vi "放置控件.vi"(8 "error in (no error)":errorcluster caption="错误输入（无错误）", 11 "程序响应 输入":refnum<class "程序响应.lvclass">) -> (0 "error out":errorcluster caption="错误输出", 3 "程序响应 输出":refnum<class "程序响应.lvclass">)   [LabVIEW 2018, in "程序响应.lvlib" / "程序响应.lvclass"]
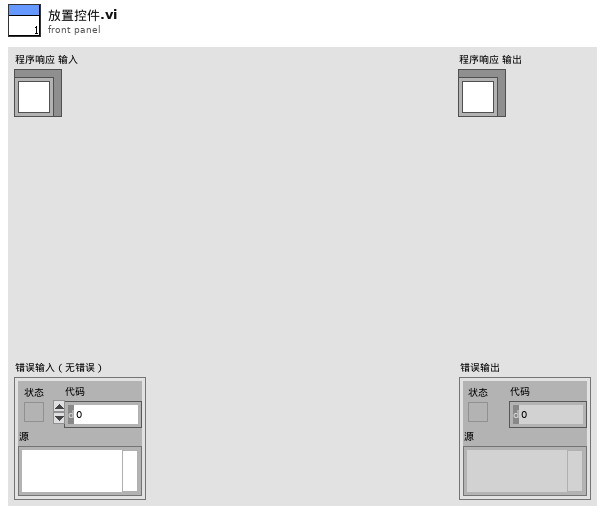
[diagram p1: front panel]
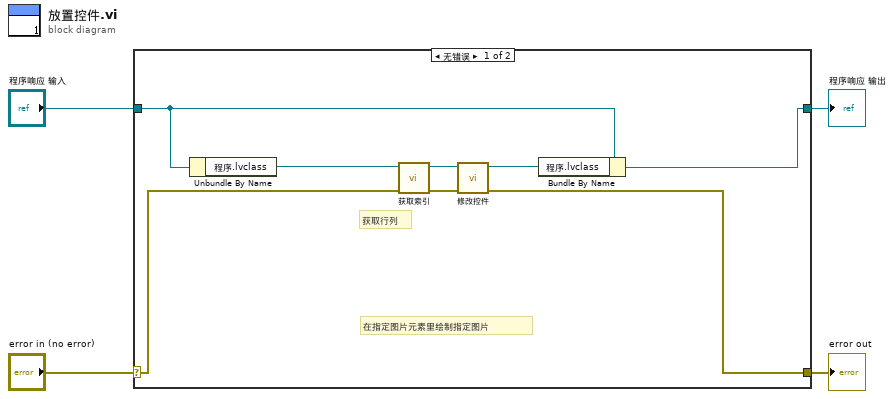
[diagram p0: block diagram]
diagram:
  n1 = case shown="无错误" "error in (no error)" {
    selector: "error in (no error)" -> [w5 w14]
    tunnel: [w9 w14] -> w3
    tunnel: [w11 w13] -> w1
    tunnel: "程序响应 输入" -> [w12 w13]
    frame No Error {
      # "在指定图片元素里绘制指定图片"
      # "获取行列"
      n2 = Unbundle By Name(w12) -> ("程序.lvclass"=w6:refnum<class "程序.lvclass">)
      n3 = call-dynamic "获取索引.vi"("error in (no error)"=w5, "程序 输入"=w6) -> ("error out"=w7:errorcluster, "程序 输出"=w8:refnum<class "程序.lvclass">)  [unwired: 8 in]
      n4 = call-dynamic "修改控件.vi"("error in (no error)"=w7, "程序 输入"=w8) -> ("error out"=w9:errorcluster, "程序 输出"=w10:refnum<class "程序.lvclass">)  [unwired: 8 in]
      n5 = Bundle By Name(cluster=w12, "程序.lvclass"=w10) -> (w11:refnum<class "程序响应.lvclass">)
    }
    frame Error {
    }
  }
  "error out" <- w3
  "程序响应 输出" <- w1
